vi "WPI_IMU_ADIS16448_Tilt_RoboBees.vi"(9 "Mag":cluster{"Xmag":dbl, "Ymag":dbl, "Zmag":dbl}, 10 "Accel":T1) -> (0 "error":bool, 1 "Yaw":dbl(knob) scale=-180.0..180.0, 2 "Roll":dbl(knob) scale=-180.0..180.0, 3 "Pitch":dbl(knob) scale=-90.0..90.0)   [LabVIEW 2015, in "Apple Pi Gyro Library.lvlib" / "FRC_ADIS16448_IMU.lvlib"]
uses:
  FRC_ADIS16448_IMU.lvlib
panel:
  in  "tol":dbl=0.05
  # "When Sensor oriented with positive X-axis\npointing forward, and positive Y-axis\npointing left, and positive Z axis pointing up :\n\nRoll is rotation about X-axis, clockwise roll,\n(looking in + X direction), is positive.\n\nPitch is rotation about Y-axis, clockwise pitch\n(looking in + Y direction), is positive.\n\nYaw is rotation about Z-axis, clockwise yaw\n(looking in + Z direction), is positive."
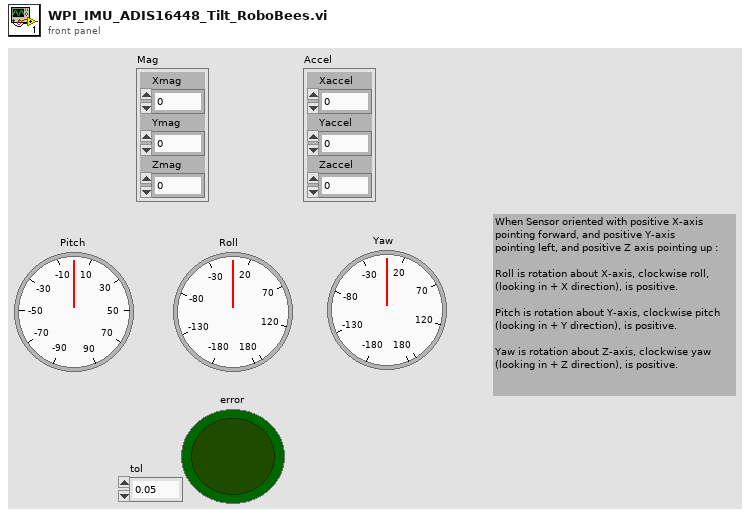
[diagram p1: front panel]
types:
  T1 = cluster{"Xaccel":dbl, "Yaccel":dbl, "Zaccel":dbl}
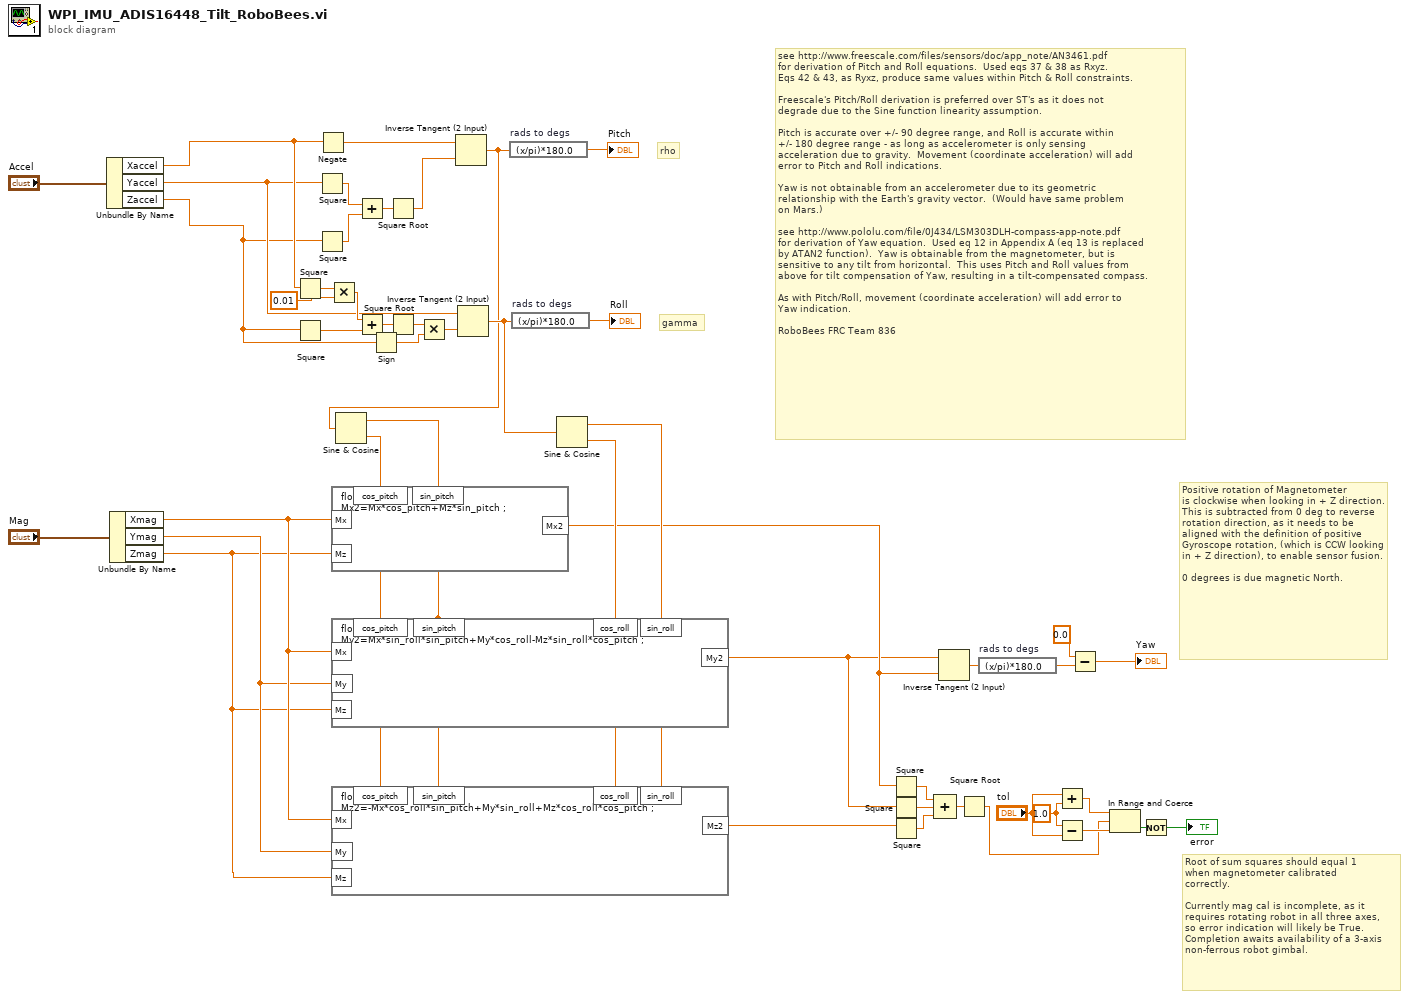
[diagram p0: block diagram]
diagram:
  w21 = 1.0 ("upper limit")
  # "Positive rotation of Magnetometer\nis clockwise when looking in + Z direction.  This is subtracted from 0 deg to reverse rotation direction, as it needs to be aligned with the definition of positive Gyroscope rotation, (which is CCW looking in + Z direction), to enable sensor fusion.\n\n0 degrees is due magnetic North."
  # "Root of sum squares should equal 1\nwhen magnetometer calibrated\ncorrectly.\n\nCurrently mag cal is incomplete, as it\nrequires rotating robot in all three axes, \nso error indication will likely be True.\nCompletion awaits availability of a 3-axis\nnon-ferrous robot gimbal."
  # "gamma"
  # "rho"
  # "see http://www.freescale.com/files/sensors/doc/app_note/AN3461.pdf\nfor derivation of Pitch and Roll equations.  Used eqs 37 & 38 as Rxyz.\nEqs 42 & 43, as Ryxz, produce same values within Pitch & Roll constraints.\n\nFreescale's Pitch/Roll derivation is preferred over ST's as it does not\ndegrade due to the Sine function linearity assumption.\n\nPitch is accurate over +/- 90 degree range, and Roll is accurate within\n+/- 180 degree range - as long as accelerometer is only sensing\nacceleration due to gravity.  Movement (coordinate acceleration) will add\nerror to Pitch and Roll indications.\n\nYaw is not obtainable from an accelerometer due to its geometric \nrelationship with the Earth's gravity vector.  (Would have same problem\non Mars.)\n\nsee http://www.pololu.com/file/0J434/LSM303DLH-compass-app-note.pdf\nfor derivation of Yaw equation.  Used eq 12 in Appendix A (eq 13 is replaced\nby ATAN2 function).  Yaw is obtainable from the magnetometer, but is\nsensitive to any tilt from horizontal.  This uses Pitch and Roll values from\nabove for tilt compensation of Yaw, resulting in a tilt-compensated compass.\n\nAs with Pitch/Roll, movement (coordinate acceleration) will add error to\nYaw indication.\n\nRoboBees FRC Team 836"
  n1 = Unbundle By Name("Accel") -> ("Xaccel"=w34:dbl, "Yaccel"=w33:dbl, "Zaccel"=w32:dbl)
  n2 = Unbundle By Name("Mag") -> ("Xmag"=w13:dbl, "Ymag"=w12:dbl, "Zmag"=w11:dbl)
  n3 = Square(x=w34) -> (x^2=w42:dbl)
  n4 = Square(x=w32) -> (x^2=w39:dbl)
  n5 = Square(x=w33) -> (x^2=w35:dbl)
  n6 = Square(x=w32) -> (x^2=w36:dbl)
  n7 = Negate(x=w34) -> (-x=w44:dbl)
  n8 = Multiply(x=w42, y=0.01 ("u 2")) -> (x*y=w43:dbl)
  n9 = Add(x=w35, y=w36) -> (x+y=w37:dbl)
  n10 = Add(x=w43, y=w39) -> (x+y=w38:dbl)
  n11 = Sign(1:w32) -> (0:w41:dbl)
  n12 = Square Root(x=w37) -> (sqrt(x)=w45:dbl)
  n13 = Square Root(x=w38) -> (sqrt(x)=w40:dbl)
  n14 = Multiply(x=w40, y=w41) -> (x*y=w46:dbl)
  n15 = Inverse Tangent (2 Input)(1:w45, 2:w44) -> (0:w4:dbl)
  n16 = Sine & Cosine(0:w4) -> (1:w30:dbl, 2:w31:dbl)
  n17 = formula code="float Mx2;\nMx2=Mx*cos_pitch+Mz*sin_pitch ;"("Mx"=w13, "cos_pitch"=w31, "sin_pitch"=w30, "Mz"=w11) -> ("Mx2"=w15:dbl)
  n18 = Inverse Tangent (2 Input)(1:w46, 2:w33) -> (0:w5:dbl)
  n19 = expression code="(x/pi)*180.0" "rads to degs"(w4) -> (→"Pitch":dbl)
  n20 = expression code="(x/pi)*180.0" "rads to degs"(w5) -> (→"Roll":dbl)
  n21 = Sine & Cosine(0:w5) -> (1:w28:dbl, 2:w29:dbl)
  n22 = formula code="float My2;\nMy2=Mx*sin_roll*sin_pitch+My*cos_roll-Mz*sin_roll*cos_pitch ;"("Mx"=w13, "cos_pitch"=w31, "sin_pitch"=w30, "Mz"=w11, "My"=w12, "sin_roll"=w28, "cos_roll"=w29) -> ("My2"=w14:dbl)
  n23 = formula code="float Mz2;\nMz2=-Mx*cos_roll*sin_pitch+My*sin_roll+Mz*cos_roll*cos_pitch ;"("Mx"=w13, "cos_pitch"=w31, "sin_pitch"=w30, "Mz"=w11, "My"=w12, "sin_roll"=w28, "cos_roll"=w29) -> ("Mz2"=w24:dbl)
  n24 = Square(x=w15) -> (x^2=w23:dbl)
  n25 = Square(x=w14) -> (x^2=w27:dbl)
  n26 = Square(x=w24) -> (x^2=w26:dbl)
  n27 = Compound Arithmetic op=ADD(w23, w27, w26) -> (w25:dbl)
  n28 = Inverse Tangent (2 Input)(1:w15, 2:w14) -> (0:w8:dbl)
  n29 = Square Root(x=w25) -> (sqrt(x)=w18:dbl)
  n30 = expression code="(x/pi)*180.0" "rads to degs"(w8) -> (w7:dbl)
  n31 = Add(x="tol", y=w21) -> (x+y=w22:dbl)
  n32 = Subtract(x=w21, y="tol") -> (x-y=w20:dbl)
  n33 = Subtract(x=0.0, y=w7) -> (x-y=→"Yaw":dbl)
  n34 = In Range and Coerce(upper limit=w22, x=w18, lower limit=w20) -> (In Range?=w19:bool)  [unwired: 1 out]
  n35 = Not(x=w19) -> (.not. x?=→"error":bool)
